vi "Convert Tooth Angles to Angles FIFO.vi"(2 "Cycle Angle?":bool, 3 "Tooth Angles":cluster{"Falling Edge":dbl, "Rising Edge":dbl}[](array[cluster])) -> (0 "First Rising?":bool, 1 "FullyCustomProfile":u64[](array[numeric]))   [LabVIEW 2011, in "Engine Sim System Explorer.lvlib"]
uses:
  Engine Sim System Explorer.lvlib
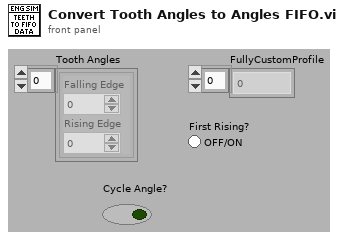
[diagram p1: front panel]
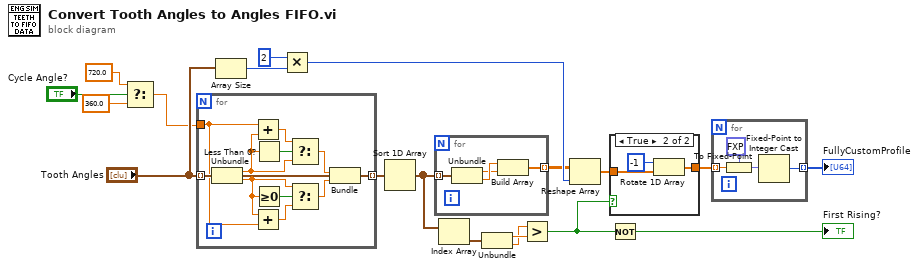
[diagram p0: block diagram]
diagram:
  n1 = Select(t=720.0 ("y"), s="Cycle Angle?", f=360.0) -> (s? t:f=w2:dbl)
  n2 = for {
    tunnel: "Tooth Angles" -> [w24] mode=indexing
    tunnel: [w21] -> w7 mode=indexing
    tunnel: w2 -> [w20]
    n3 = Unbundle(w24) -> ("Falling Edge"=w27:dbl, "Rising Edge"=w25:dbl)
    n4 = Add(x=w20, y=w27) -> (x+y=w28:dbl)
    n5 = Add(x=w25, y=w20) -> (x+y=w26:dbl)
    n6 = Less Than 0?(x=w27) -> (x < 0?=w30:bool)
    n7 = Greater Or Equal To 0?(x=w25) -> (x >= 0?=w29:bool)
    n8 = Select(t=w28, s=w30, f=w27) -> (s? t:f=w23:dbl)
    n9 = Select(t=w25, s=w29, f=w26) -> (s? t:f=w22:dbl)
    n10 = Bundle(cluster=w24, "Falling Edge"=w23, "Rising Edge"=w22) -> (w21:cluster{"Falling Edge":dbl, "Rising Edge":dbl})
  }
  n11 = Array Size(array="Tooth Angles") -> (size(s)=w18:i32)
  n12 = Multiply(x=u16 2, y=w18) -> (x*y=w19:i32)
  n13 = Sort 1D Array(array=w7) -> (sorted array=w9:cluster{"Falling Edge":dbl, "Rising Edge":dbl}[])
  n14 = for {
    tunnel: w9 -> [w34] mode=indexing
    tunnel: [w31] -> w8 mode=indexing
    n15 = Unbundle(w34) -> ("Falling Edge"=w32:dbl, "Rising Edge"=w33:dbl)
    n16 = Build Array(w33, w32) -> (w31:dbl[])
  }
  n17 = Index Array(array=w9) -> (element=w10:cluster{"Falling Edge":dbl, "Rising Edge":dbl})  [unwired: 1 in]
  n18 = Unbundle(w10) -> ("Falling Edge"=w12:dbl, "Rising Edge"=w11:dbl)
  n19 = Greater?(x=w11, y=w12) -> (0:w14:bool)
  n20 = Reshape Array(w8, w19) -> (w13:dbl[])
  n21 = case shown="True" w14 {
    tunnel: w13 -> [w35 w38]
    tunnel: [w35 w36] -> w6
    frame False {
    }
    frame True {
      n22 = Rotate 1D Array(1:w38, 2:-1 ("n")) -> (0:w36:dbl[])
    }
  }
  n23 = Not(x=w14) -> (.not. x?=→"First Rising?":bool)
  n24 = for {
    tunnel: w6 -> [w42] mode=indexing
    tunnel: [w39] -> w5 mode=indexing
    n25 = To Fixed-Point(fixed-point type=fxp<+,61,10> 0.0 ("Element"), number=w42) -> (fixed-point=w40:fxp<+,61,10>)
    n26 = Fixed-Point to Integer Cast(1:w40) -> (0:w39:u64)
  }
  "FullyCustomProfile" <- w5
